vi "create.OrderExecutedAtPriceSize.vi"(11 "OrderExecutedAtPriceSize.Parameters":T1={"Time Offset"=447000, "Order Id"="ORID0001", "Executed Quantity"=20000, "Execution Id"="AAPL", "Remaining Quantity"=20000, "Price"=0.905}) -> (2 "Bytes.Out":u8[](array[numeric]) format="%.0x", 3 "MessageBase out":refnum<class "OrderExecutedAtPriceSize.lvclass">)   [LabVIEW 2022 SP3]
uses:
  OrderExecuted/OrderExecutedAtPriceSize.Parameters.ctl
  OrderExecuted/OrderExecutedAtPriceSize.lvclass
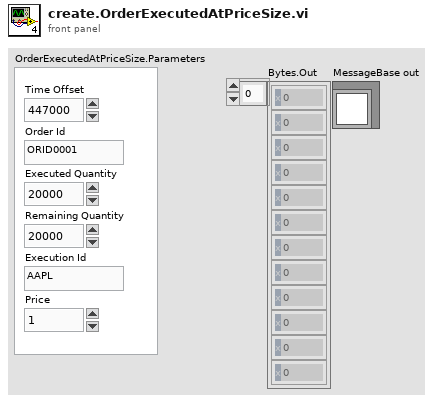
[diagram p1: front panel]
types:
  T1 = typedef "OrderExecutedAtPriceSize.lvclass/OrderExecutedAtPriceSize.Parameters.ctl" = cluster{"Time Offset":u32, "Order Id":string, "Executed Quantity":u32, "Execution Id":string, "Remaining Quantity":u32, "Price":dbl}
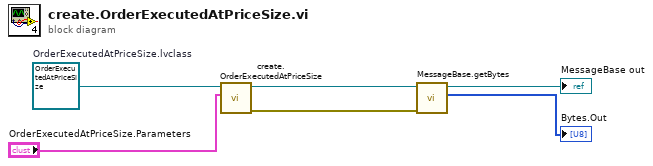
[diagram p0: block diagram]
diagram:
  w5 = refnum<class "OrderExecutedAtPriceSize.lvclass"> refnum  # OrderExecutedAtPriceSize.lvclass
  n1 = call-dynamic "create.OrderExecutedAtPriceSize.vi"("OrderExecutedAtPriceSize.Parameters"="OrderExecutedAtPriceSize.Parameters", "OrderExecutedAtPriceSize in"=w5) -> ("error out"=w3:errorcluster, "OrderExecutedAtPriceSize out"=w2:refnum<class "OrderExecutedAtPriceSize.lvclass">)  [unwired: 8 in]
  n2 = call-dynamic "MessageBase.getBytes.vi"("error in (no error)"=w3, "MessageBase in"=w2) -> ("Bytes.out"=→"Bytes.Out":u8[], "MessageBase out"=→"MessageBase out":refnum<class "OrderExecutedAtPriceSize.lvclass">)  [unwired: 7 in, 1 out]
